vi "DetermineHeadingRegime.vi"(9 "Altered regime boundaries":T1=[0, 70, 140, 220, 190, 290], 10 "Robot Heading (deg)":dbl, 11 "Trusted Absolute Wind Data (deg)":dbl) -> (3 "Sailing Regime":T2)   [LabVIEW 2013]
doc: "This VI looks at the wind and the given heading and determines which boat regime the heading is, ignoring whether or not the boat should be in a transition. It ignores the transistions because another section of the code checks whether we are in a transition and does that based on that last commanded regime, not based on the current absolute wind vs. heading of the robot. For example, if the given heading is pointed at 90 degrees (up) and the wind is from 180 degrees (left), then that heading should fall in the 'Reach - Port Tack' regime. Diagram found in\n https://docs.google.com/file/d/0B6St7IDGiYunU3FLWTZHTUFHWHc/edit\n\nEric Schneider, Feb. 2014"
uses:
  Data/TypeDefs/Sailing Regimes.ctl
  Data/TypeDefs/Regime Boundaries.ctl
  Utilities/Math/Angles/Angle/Angle.lvclass
panel:
  out "Numeric":i32
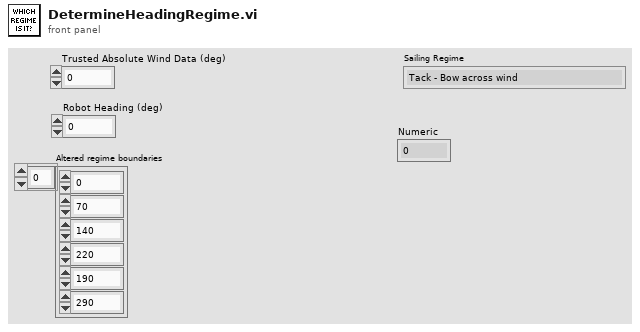
[diagram p1: front panel]
types:
  T1 = typedef "Regime Boundaries.ctl" = i32[]
  T2 = typedef "Sailing Regimes.ctl" = enum16{"Tack - Bow across wind", "Upwind - Port Tack", "Turn between Upwind/Reach - Port Tack", "Reach - Port Tack", "Turn between Reach/Run - Port Tack", "Run - Port Tack", "Jibe - Stern across wind", "Run - Starboard Tack", "Turn between Reach/Run - Starboard Tack", "Reach - Starboard Tack", "Turn between Upwind/Reach - Starboard Tack", "Upwind - Starboard Tack"}
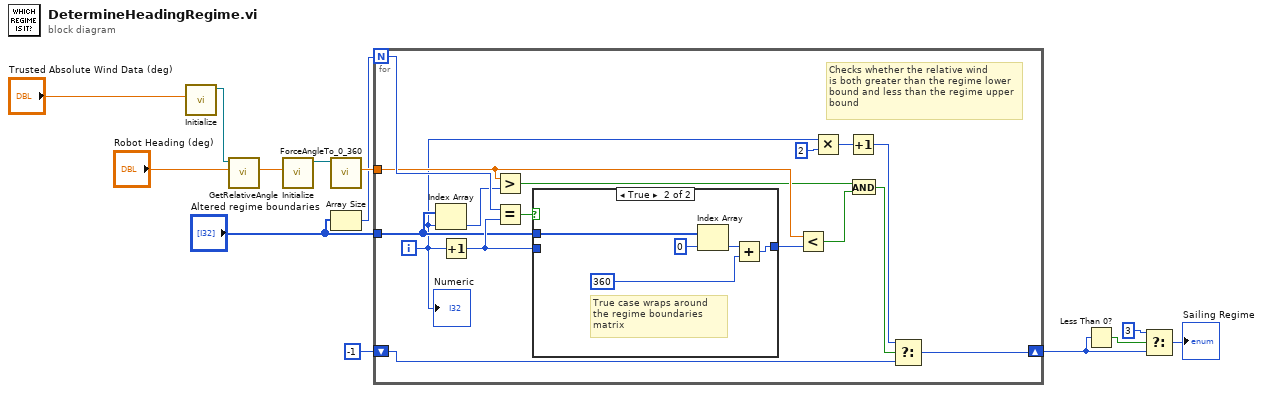
[diagram p0: block diagram]
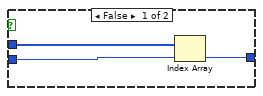
[diagram p2: hidden frame]
diagram:
  n1 = call "Initialize.vi"("Input Angle (Deg.)"="Trusted Absolute Wind Data (deg)") -> ("Angle out"=w12:refnum<class "Angle.lvclass">)  [unwired: 9 in, 1 out]
  n2 = call "GetRelativeAngle.vi"("Boat Heading (Deg.)"="Robot Heading (deg)", "Angle in"=w12) -> ("Relative Angle"=w9:dbl)  [unwired: 8 in, 1 out]
  n3 = call "Initialize.vi"("Input Angle (Deg.)"=w9) -> ("Angle out"=w8:refnum<class "Angle.lvclass">)  [unwired: 9 in, 1 out]
  n4 = call "ForceAngleTo_0_360.vi"("Angle in"=w8) -> ("Relative Angle"=w7:dbl)  [unwired: 9 in, 1 out]
  n5 = Array Size(array="Altered regime boundaries") -> (size(s)=w1:i32)
  n6 = for {
    N: w1 -> [w29]
    tunnel: "Altered regime boundaries" -> [w19]
    tunnel: w7 -> [w20]
    shift-right: [w22] -> w4
    shift-left: -1 -> [w23]
    i -> [w18]
    # "Checks whether the relative wind\nis both greater than the regime lower bound and less than the regime upper bound"
    n7 = Index Array(array=w19, index=w18) -> (element=w17:i32)
    n8 = Increment(x=w18) -> (x+1=w27:i32)
    n9 = Greater?(x=w20, y=w17) -> (0:w16:bool)
    n10 = Equal?(x=w29, y=w27) -> (x = y?=w21:bool)
    n11 = case shown="True" w21 {
      tunnel: w19 -> [w32 w37]
      tunnel: [w30 w33] -> w28
      tunnel: w27 -> [w31 _]
      frame False {
        n12 = Index Array(array=w32, index=w31) -> (element=w30:i32)
      }
      frame True {
        # "True case wraps around the regime boundaries matrix"
        n13 = Index Array(array=w37, index=0) -> (element=w35:i32)
        n14 = Add(x=w35, y=360) -> (x+y=w33:i32)
      }
    }
    n15 = Less?(x=w20, y=w28) -> (x < y?=w15:bool)
    n16 = Multiply(x=w18, y=2) -> (x*y=w26:i32)
    n17 = Increment(x=w26) -> (x+1=w25:i32)
    n18 = And(x=w16, y=w15) -> (x .and. y?=w14:bool)
    n19 = Select(t=w25, s=w14, f=w23) -> (s? t:f=w22:i32)
    "Numeric" <- w18
  }
  n20 = Less Than 0?(x=w4) -> (x < 0?=w5:bool)
  n21 = Select(t=3, s=w5, f=w4) -> (s? t:f=→"Sailing Regime":i32)
